vi "Test_PromoteElement_PromoteOK.vi"(8 "error in (no error)":errorcluster, 11 "TestCase in":refnum<class "TestArrayExtensions.lvclass">) -> (0 "error out":errorcluster, 3 "TestCase out":refnum<class "TestArrayExtensions.lvclass">)   [LabVIEW 2015, in "ArrayExtensions.lvlib" / "TestArrayExtensions.lvclass"]
uses:
  TestArrayExtensions.lvclass
  Promote Element (I32).vi
  <vilib>/addons/_JKI Toolkits/VI Tester/TestCase.llb/TestCase.lvclass
  ArrayExtensions.lvlib
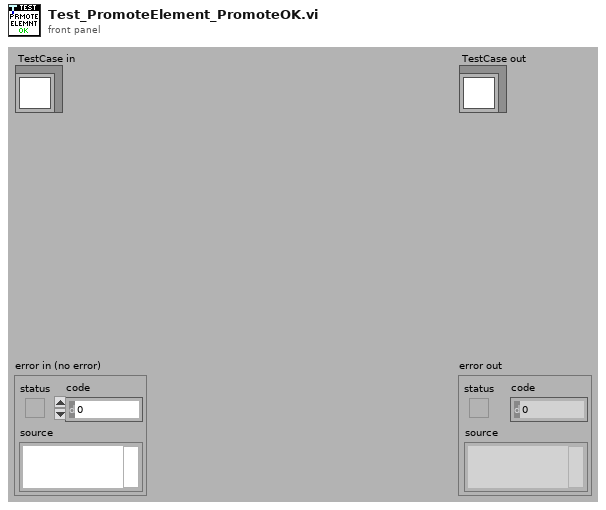
[diagram p1: front panel]
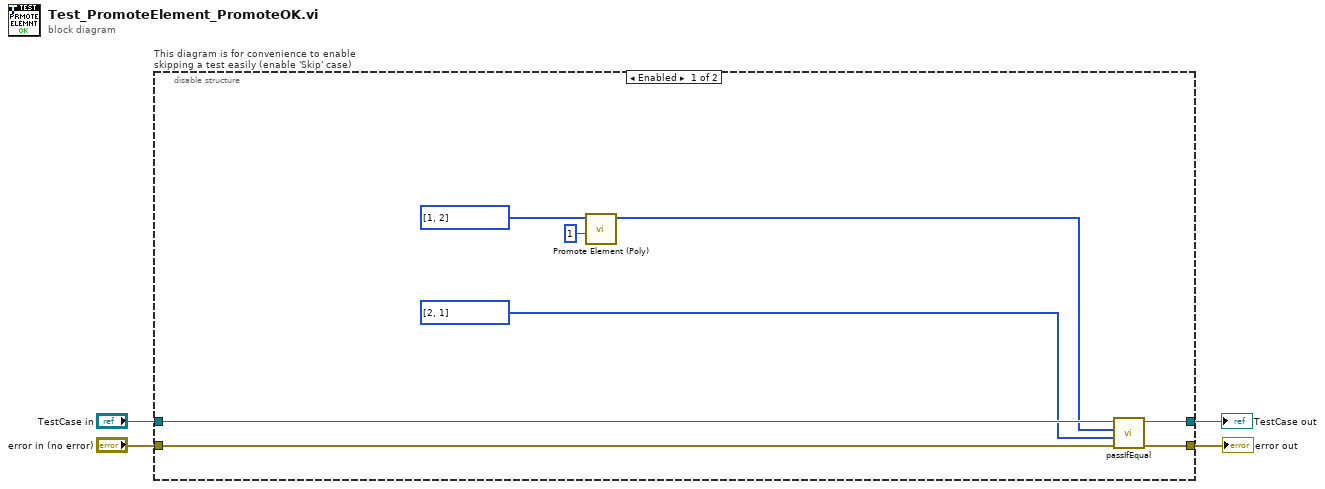
[diagram p0: block diagram]
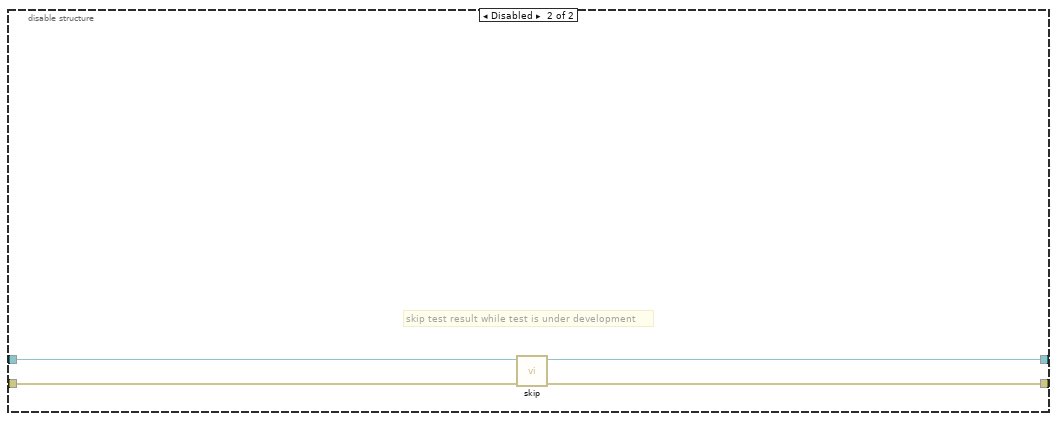
[diagram p2: hidden frame]
diagram:
  n1 = disable-structure "This diagram is for convenience to enable skipping a test easily (enable 'Skip' case)" shown="Enabled" {
    disable-tunnel: "TestCase in" -> [w12 w16]
    disable-tunnel: [w11 w14] -> w1
    disable-tunnel: [w10 w15] -> w3
    disable-tunnel: "error in (no error)" -> [w9 w13]
    frame Enabled {
      n2 = call-poly "Promote Element (Poly).vi"("Index to Promote"=1, "Array In"=i32[] [1, 2]) -> ("Array Out"=w7:i32[])  [unwired: 9 in]
      n3 = call-dynamic "passIfEqual.vi"("error in (no error)"=w9, "y"=i32[] [2, 1], "x"=w7, "TestCase in"=w12) -> ("error out"=w10:errorcluster, "TestCase out"=w11:refnum<class "TestArrayExtensions.lvclass">)  [unwired: 6 in]
    }
    frame Disabled {
      # "skip test result while test is under development"
      n4 = call <vilib>:"skip.vi"("error in (no error)"=w13, "TestCase in"=w16) -> ("error out"=w15:errorcluster, "TestCase out"=w14:refnum<class "TestArrayExtensions.lvclass">)  [unwired: 8 in]
    }
  }
  "error out" <- w3
  "TestCase out" <- w1
